vi "Remove Header.vi"(8 "error in":errorcluster, 10 "header":string, 11 "advanced-http-client in":refnum<class "advanced-http-client.lvclass">) -> (0 "error out":errorcluster, 3 "advanced-http-client out":refnum<class "advanced-http-client.lvclass">)   [LabVIEW 2020, in "advanced-http-client.lvclass"]
uses:
  advanced-http-client.lvclass
  advanced-http-client.lvclass/advanced-http-client.ctl
  <vilib>/NI/Advanced HTTP Client/Session.lvclass
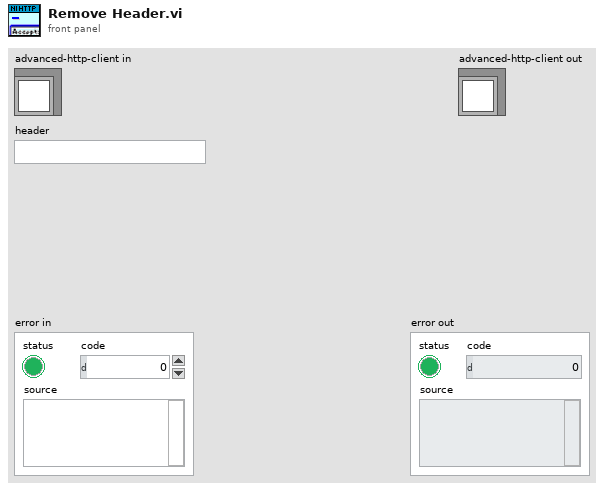
[diagram p1: front panel]
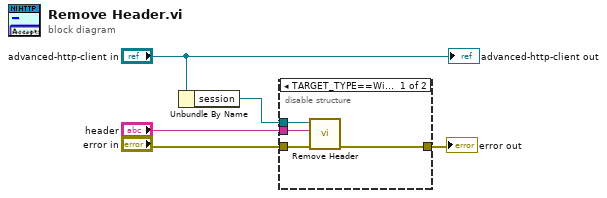
[diagram p0: block diagram]
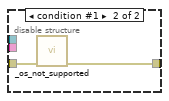
[diagram p2: hidden frame]
diagram:
  n1 = Unbundle By Name("advanced-http-client in") -> ("session"=w1:refnum<class "Session.lvclass">)
  n2 = disable-structure shown="TARGET_TYPE==Windows" {
    disable-tunnel: "error in" -> [w9 w11]
    disable-tunnel: [w8 w10] -> w4
    disable-tunnel: "header" -> [w7 _]
    disable-tunnel: w1 -> [w6 _]
    frame condition #0 (active) {
      n3 = call <vilib>:"Remove Header.vi"("error in"=w9, "header"=w7, "session in"=w6) -> ("error out"=w8:errorcluster)  [unwired: 7 in, 1 out]
    }
    frame condition #1 {
      n4 = call "_os_not_supported.vi"("error in (no error)"=w11) -> ("error out"=w10:errorcluster)  [unwired: 9 in, 1 out]
    }
  }
  "error out" <- w4
  "advanced-http-client out" <- "advanced-http-client in"
